vi "Build Bulk Create.vi"(8 "error in (no error)":errorcluster, 9 "tableName":string, 10 "DynamicParameters in":refnum<class "DynamicParameters.lvclass">[](array[class]), 11 "DbConnection in":refnum<class "DbConnection.lvclass">) -> (0 "error out":errorcluster, 2 "BulkInsertQuery":string, 3 "DbConnection out":refnum<class "DbConnection.lvclass">)   [LabVIEW 2020, in "ORM.lvlib" / "DbConnection.lvclass"]
uses:
  DbConnection.lvclass
  DynamicParameters/DynamicParameters.lvclass
  DbConnection.lvclass/DbConnection.ctl
  DynamicParameters/DynamicParameters.lvclass/DynamicParameters.ctl
  DynamicParameters/Read ParameterNames.vi
  DynamicParameters/Read FieldNames.vi
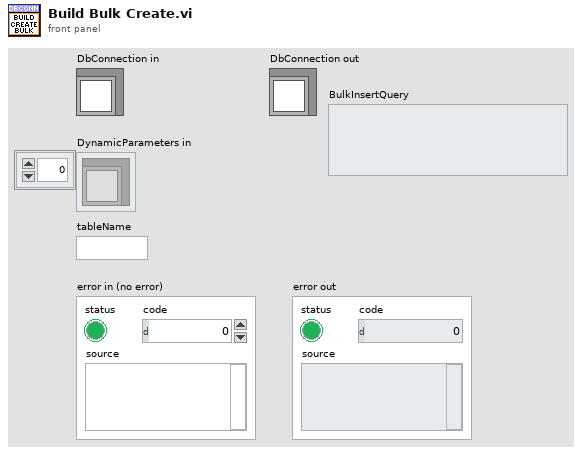
[diagram p1: front panel]
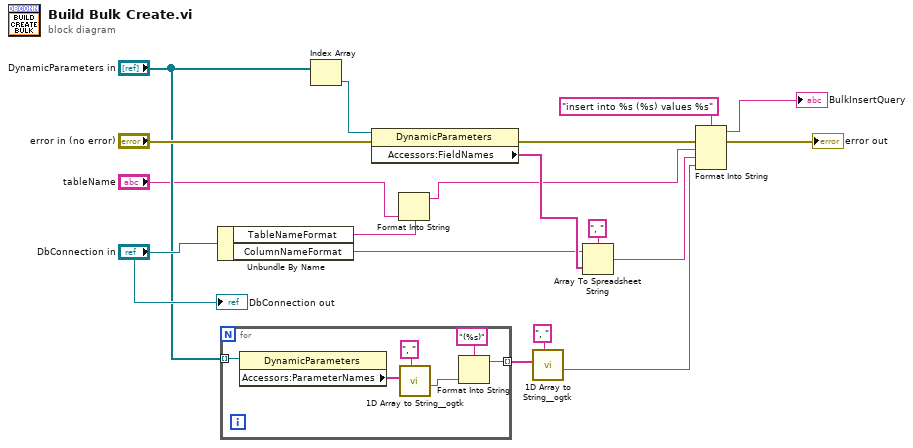
[diagram p0: block diagram]
diagram:
  n1 = Unbundle By Name("DbConnection in") -> ("TableNameFormat"=w3:string, "ColumnNameFormat"=w16:string)
  n2 = for {
    tunnel: "DynamicParameters in" -> [w23] mode=indexing
    tunnel: [w19] -> w5 mode=indexing
    n3 = property class="DynamicParameters"(reference=w23) -> ("Accessors:ParameterNames"=w22:string[])  [unwired: 1 in, 2 out]
    n4 = call <userlib>:"1D Array to String__ogtk.vi"("delimiter (Tab)"=", ", "Array of Strings"=w22) -> ("delimited string"=w21:string)  [unwired: 9 in]
    n5 = Format Into String(format string="(%s)", w21) -> (resulting string=w19:string)  [unwired: 2 in, 1 out]
  }
  n6 = Index Array(array="DynamicParameters in") -> (element=w8:refnum<class "DynamicParameters.lvclass">)  [unwired: 1 in]
  n7 = property class="DynamicParameters"(reference=w8, error in="error in (no error)") -> (error out=w13:errorcluster, "Accessors:FieldNames"=w18:string[])  [unwired: 1 out]
  n8 = Format Into String(format string=w3, "tableName") -> (resulting string=w1:string)  [unwired: 2 in, 1 out]
  n9 = call <userlib>:"1D Array to String__ogtk.vi"("delimiter (Tab)"=", ", "Array of Strings"=w5) -> ("delimited string"=w4:string)  [unwired: 9 in]
  n10 = Array To Spreadsheet String(delimiter (Tab)=", ", array=w18, 3:w16) -> (spreadsheet string=w12:string)
  n11 = Format Into String(format string="insert into %s (%s) values %s", error in=w13, w1, w12, w4) -> (resulting string=→"BulkInsertQuery":string, error out=→"error out":errorcluster)  [unwired: 1 in]
  "DbConnection out" <- "DbConnection in"
